vi "average test.vi"() -> ()   [LabVIEW 2013]
panel:
  out "output cluster":cluster{dbl[]}
  in  "Average":i32
  out "OKH":bool
  in  "’âŽ~":bool=TRUE
  out "XY Graph":cluster{dbl[], dbl[]}(graph) caption="pixel vs A/D Counts"
  in  "Pixel":u16=1024
  out "OKH 2":bool
  out "PipeHandle":i32=-1
  out "DeviceHandle":i32=-1
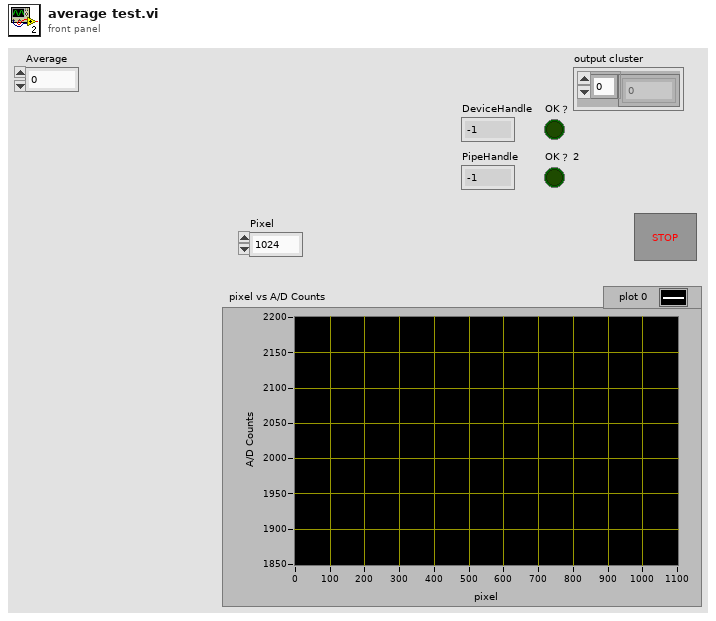
[diagram p1: front panel]
types:
  T1 = typedef "specu1a 1.0.0 Product Information.ctl" = cluster{"UnitID":string, "Sensor Name":string, "Serial Number":string, "Reserved":string, "Wave Upper":u16, "Wave Lower":u16}
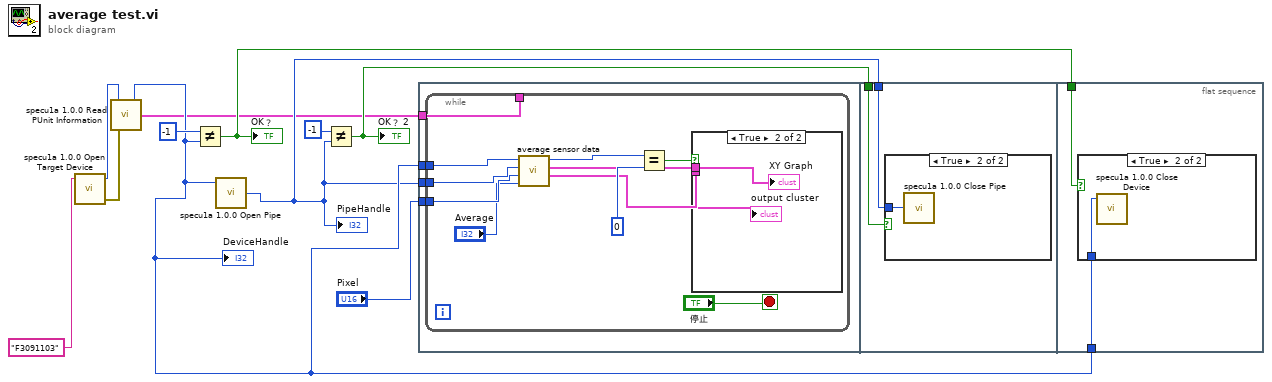
[diagram p0: block diagram]
diagram:
  n1 = call <instrlib>:"specu1a 1.0.0 Open Target Device.vi"("Unit ID"="F3091103") -> ("error out"=w4:errorcluster, "Device Handle"=w5:i32)  [unwired: 2 in, 1 out]
  n2 = call <instrlib>:"specu1a 1.0.0 Read PUnit Information.vi"("error in (no error)"=w4, "Device Handle"=w5) -> ("Unit Information out"=w1:T1, "Device Handle out"=w3:i32)  [unwired: 1 in, 1 out]
  "DeviceHandle" <- w3
  n3 = Not Equal?(x=-1, y=w3) -> (x != y?=w9:bool)
  "OKH" <- w9
  n4 = call <instrlib>:"specu1a 1.0.0 Open Pipe.vi"("Device Handle"=w3) -> ("Pipe Handle"=w2:i32)  [unwired: 2 in, 2 out]
  "PipeHandle" <- w2
  n5 = Not Equal?(x=-1, y=w2) -> (x != y?=w8:bool)
  "OKH 2" <- w8
  n6 = flat-sequence {
    tunnel: w3 -> [w15]
    tunnel: w2 -> [w14]
    tunnel: "Pixel" -> [w13]
    tunnel: w1 -> [w12]
    tunnel: w8 -> [w29]
    tunnel: w2 -> [w28]
    tunnel: w3 -> [w32]
    tunnel: w9 -> [w31]
    frame #0 {
      n7 = while {
        tunnel: w15 -> [w21]
        tunnel: w14 -> [w20]
        tunnel: w13 -> [w19]
        tunnel: w12 -> [_]
        stop <- "’âŽ~" stop-if-true
        n8 = call <instrlib>:"average sensor data.vi"("Numeric"="Average", "PixelSize"=w19, "Pipe handle"=w20, "Device Handle 2"=w21) -> ("output cluster"=w18:cluster{dbl[]}, "XY Graph"=w16:cluster{dbl[], dbl[]}, "return type"=w22:u16)  [unwired: 5 in]
        n9 = Equal?(x=w22, y=0) -> (x = y?=w25:bool)
        n10 = case shown="True" w25 {
          tunnel: w18 -> [_ w26]
          tunnel: w16 -> [_ w27]
          frame False {
          }
          frame True {
            "XY Graph" <- w27
            "output cluster" <- w26
          }
        }
      }
    }
    frame #1 {
      n11 = case shown="True" w29 {
        tunnel: w28 -> [_ w30]
        frame False {
        }
        frame True {
          n12 = call <instrlib>:"specu1a 1.0.0 Close Pipe.vi"("Pipe Handle"=w30) -> ()  [unwired: 3 in, 2 out]
        }
      }
    }
    frame #2 {
      n13 = case shown="True" w31 {
        tunnel: w32 -> [_ w33]
        frame False {
        }
        frame True {
          n14 = call <instrlib>:"specu1a 1.0.0 Close Device.vi"("Device Handle"=w33) -> ()  [unwired: 4 in, 1 out]
        }
      }
    }
  }
